vi "udp_receive_py.vi"() -> ()   [LabVIEW 2020]
panel:
  out "*(타입 *) &x":u32
  out "Numeric 4":dbl
  in  "send object cluster":T1
  in  "stop 2":bool
  out "Rz":sgl
  out "Ry":sgl
  out "Rx":sgl
  out "z":sgl
  out "y":sgl
  out "x":sgl
  out "error":sgl
  out "function":sgl
  out "string":string
  in  "stop":bool
  out "Numeric":i32
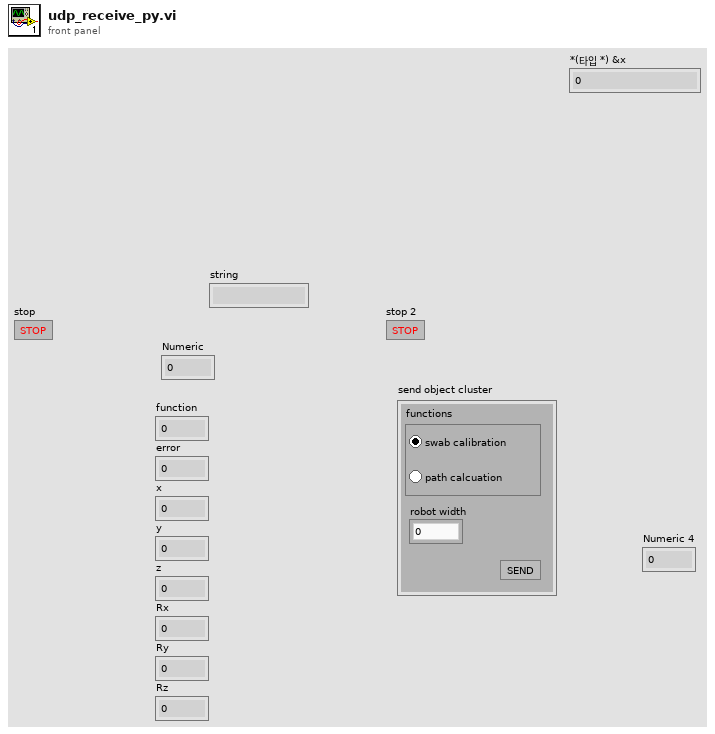
[diagram p1: front panel]
types:
  T1 = cluster{"functions":enum32{"swab calibration", "path calculation"}, "robot width":sgl, "send":bool}
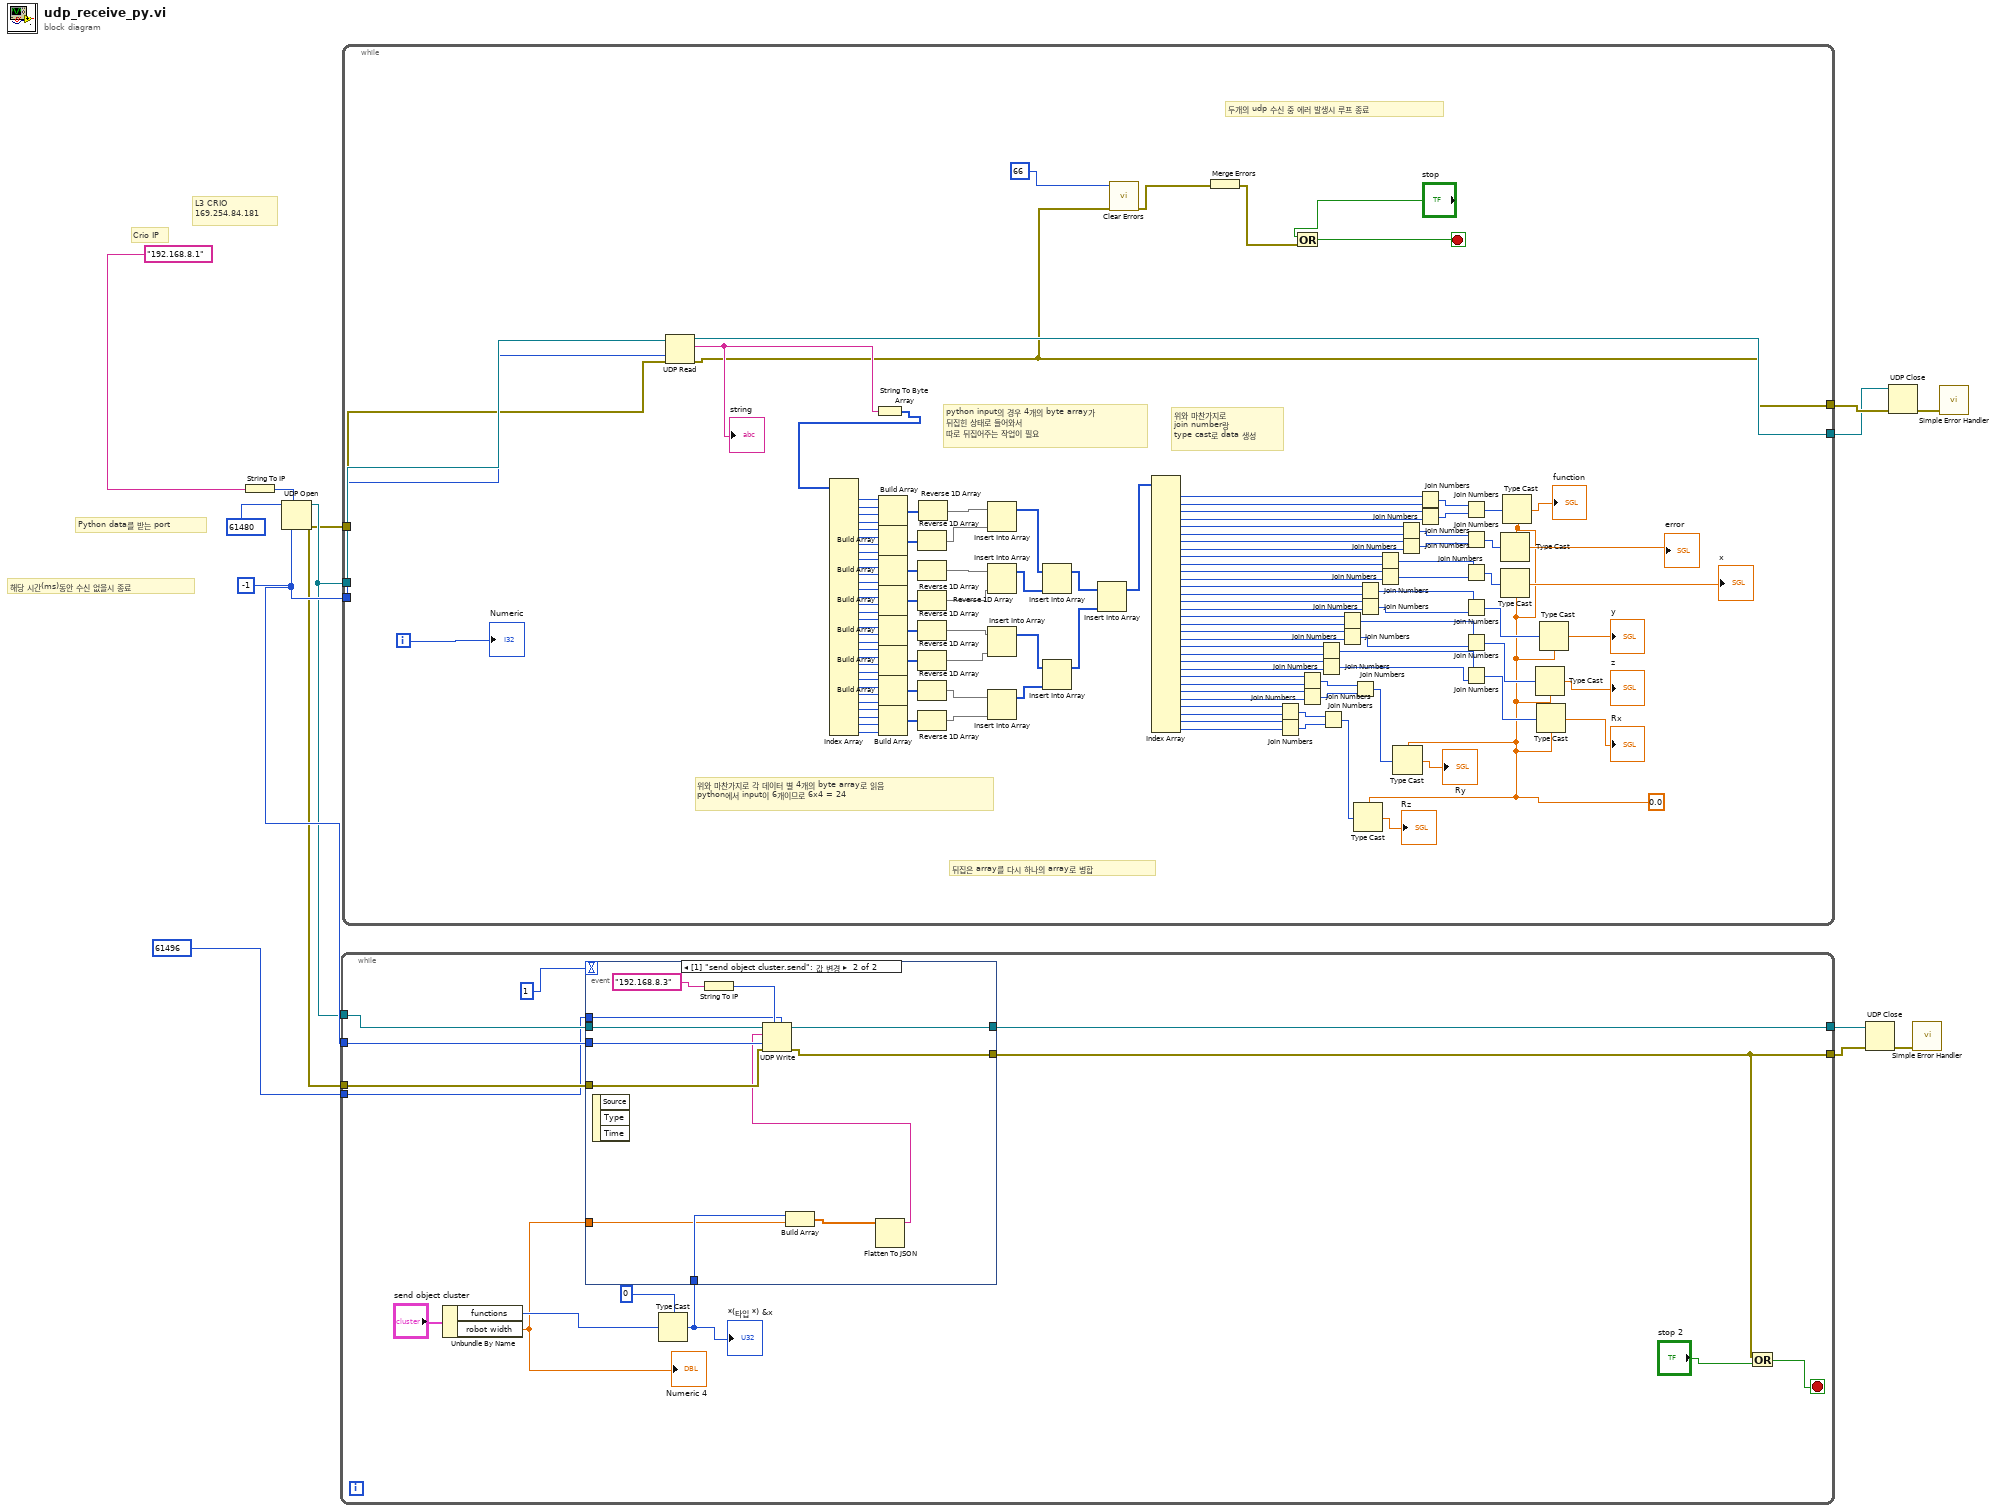
[diagram p0: block diagram]
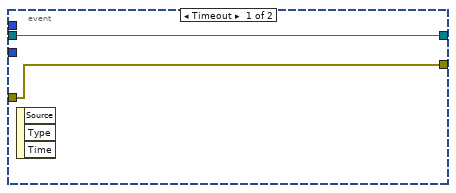
[diagram p2: hidden frame]
diagram:
  w5 = -1 ("timeout ms (25000)")
  # "L3 CRIO\n169.254.84.181"
  # "해당 시간(ms)동안 수신 없을시 종료"
  # "Crio IP"
  # "Python data를 받는 port"
  n1 = String To IP(1:"192.168.8.1" ("service name")) -> (0:w12:u32)
  n2 = UDP Open(7:w12, 9:w5, 11:u16 61480 ("port")) -> (port=w4:refnum<k16>, 0:w3:errorcluster)  [unwired: 2 in, 1 out]
  n3 = while {
    tunnel: w4 -> [w27]
    tunnel: w5 -> [w26]
    tunnel: w3 -> [w25]
    tunnel: [w24] -> w8
    tunnel: [w23] -> w7
    tunnel: u16 61496 ("port") -> [w19]
    stop <- w22 stop-if-true
    n4 = Unbundle By Name("send object cluster") -> ("functions"=w16:enum32{"swab calibration", "path calculation"}, "robot width"=w14:sgl)
    "Numeric 4" <- w14
    n5 = Type Cast(type=u32 0, x=w16) -> (*(type *) &x=w15:u32)
    "*(타입 *) &x" <- w15
    n6 = event shown="[1] \"send object cluster.send\": 값 변경" {
      selector: _ -> [_ _]
      dyn-events: _ -> [_ _]
      timeout: 1 ("timeout ms (25000)") -> [_ _]
      tunnel: w27 -> [w29 w41]
      tunnel: w26 -> [_ w40]
      tunnel: w25 -> [w28 w39]
      tunnel: [w29 w36] -> w24
      tunnel: [w28 w35] -> w23
      tunnel: w19 -> [_ w34]
      tunnel: w15 -> [_ w32]
      tunnel: w14 -> [_ w31]
      event Timeout {
        n7 = event-data() -> ()  [unwired: 1 in, 3 out]
      }
      event "send object cluster.send": Value Change {
        n8 = event-data() -> ()  [unwired: 1 in, 3 out]
        n9 = String To IP(1:"192.168.8.3" ("service name")) -> (0:w37:u32)
        n10 = Build Array(w32, w31) -> (w33:sgl[])
        n11 = Flatten To JSON(anything=w33) -> (JSON string=w30:string)  [unwired: 2 in, 1 out]
        n12 = UDP Write(address=w37, port or service name=w34, connection ID=w41, data in=w30, 8:w39, 9:w40) -> (error out=w35:errorcluster, 3:w36:refnum<k16>)
      }
    }
    n13 = Or(x=w23, y="stop 2") -> (x .or. y?=w22:bool)
  }
  n14 = while {
    tunnel: w4 -> [w171]
    tunnel: w5 -> [w170]
    tunnel: w3 -> [w169]
    tunnel: [w44] -> w11
    tunnel: [w168] -> w10
    i -> [w174]
    stop <- w172 stop-if-true
    w47 = sgl 0.0
    # "두개의 udp 수신 중 에러 발생시 루프 종료"
    # "위와 마찬가지로\njoin number랑\ntype cast로 data 생성"
    # "뒤집은 array를 다시 하나의 array로 병합"
    # "python input의 경우 4개의 byte array가\n뒤집힌 상태로 들어와서\n따로 뒤집어주는 작업이 필요"
    # "위와 마찬가지로 각 데이터 별 4개의 byte array로 읽음\npython에서 input이 6개이므로 6x4 = 24"
    n15 = UDP Read(connection ID=w171, timeout ms (25000)=w170, 8:w169) -> (data out=w131:string, error out=w44:errorcluster, 3:w168:refnum<k16>)  [unwired: 1 in, 2 out]
    "string" <- w131
    n16 = String To Byte Array(string=w131) -> (unsigned byte array=w165:u8[])
    n17 = Index Array(array=w165) -> (element #1=w166:u8, element #2=w164:u8, element #3=w163:u8, element #4=w162:u8, element #5=w161:u8, element #6=w160:u8, element #7=w159:u8, element #8=w158:u8, element #9=w157:u8, element #10=w156:u8, element #11=w155:u8, element #12=w154:u8, element #13=w130:u8, element #14=w129:u8, element #15=w128:u8, element #16=w127:u8, element #17=w126:u8, element #18=w125:u8, element #19=w124:u8, element #20=w123:u8, element #21=w122:u8, element #22=w121:u8, element #23=w120:u8, element #24=w119:u8, element #25=w88:u8, element #26=w87:u8, element #27=w86:u8, element #28=w85:u8, element #29=w84:u8, element #30=w83:u8, element #31=w82:u8, element #32=w81:u8)  [unwired: 32 in]
    n18 = Build Array(w166, w164, w163, w162) -> (w153:u8[])
    n19 = Build Array(w161, w160, w159, w158) -> (w152:u8[])
    n20 = Build Array(w157, w156, w155, w154) -> (w151:u8[])
    n21 = Build Array(w130, w129, w128, w127) -> (w118:u8[])
    n22 = Build Array(w126, w125, w124, w123) -> (w117:u8[])
    n23 = Build Array(w122, w121, w120, w119) -> (w116:u8[])
    n24 = Build Array(w88, w87, w86, w85) -> (w80:u8[])
    n25 = Build Array(w84, w83, w82, w81) -> (w79:u8[])
    n26 = Reverse 1D Array(array=w152) -> (reversed array=w149:u8[])
    n27 = Reverse 1D Array(array=w151) -> (reversed array=w115:u8[])
    n28 = Reverse 1D Array(array=w118) -> (reversed array=w114:u8[])
    n29 = Reverse 1D Array(array=w117) -> (reversed array=w113:u8[])
    n30 = Reverse 1D Array(array=w116) -> (reversed array=w112:u8[])
    n31 = Reverse 1D Array(array=w80) -> (reversed array=w78:u8[])
    n32 = Reverse 1D Array(array=w79) -> (reversed array=w77:u8[])
    n33 = Reverse 1D Array(array=w153) -> (reversed array=w150:u8[])
    n34 = Insert Into Array(array=w150, new element=w149) -> (w74:u8[])  [unwired: 1 in]
    n35 = Insert Into Array(array=w115, new element=w114) -> (w73:u8[])  [unwired: 1 in]
    n36 = Insert Into Array(array=w113, new element=w112) -> (w75:u8[])  [unwired: 1 in]
    n37 = Insert Into Array(array=w78, new element=w77) -> (w76:u8[])  [unwired: 1 in]
    n38 = Insert Into Array(array=w74, new element=w73) -> (w72:u8[])  [unwired: 1 in]
    n39 = Insert Into Array(array=w75, new element=w76) -> (w71:u8[])  [unwired: 1 in]
    n40 = Insert Into Array(array=w72, new element=w71) -> (w148:u8[])  [unwired: 1 in]
    n41 = call <vilib>:"Clear Errors.vi"("error in (no error)"=w44, "specific error code to clear (0: all)"=66) -> ("error out"=w43:errorcluster)  [unwired: 4 in, 1 out]
    n42 = Index Array(array=w148) -> (element #1=w146:u8, element #2=w145:u8, element #3=w144:u8, element #4=w143:u8, element #5=w142:u8, element #6=w98:u8, element #7=w147:u8, element #8=w97:u8, element #9=w141:u8, element #10=w94:u8, element #11=w93:u8, element #12=w92:u8, element #13=w107:u8, element #14=w91:u8, element #15=w90:u8, element #16=w89:u8, element #17=w70:u8, element #18=w69:u8, element #19=w68:u8, element #20=w67:u8, element #21=w106:u8, element #22=w65:u8, element #23=w64:u8, element #24=w63:u8, element #25=w61:u8, element #26=w60:u8, element #27=w59:u8, element #28=w58:u8, element #29=w57:u8, element #30=w56:u8, element #31=w55:u8, element #32=w54:u8)  [unwired: 32 in]
    n43 = Merge Errors(w43) -> (w167:errorcluster)
    n44 = Join Numbers(hi=w57, lo=w56) -> ((hi.lo)=w53:u16)
    n45 = Join Numbers(hi=w55, lo=w54) -> ((hi.lo)=w52:u16)
    n46 = Or(x="stop", y=w167) -> (x .or. y?=w172:bool)
    n47 = Join Numbers(hi=w61, lo=w60) -> ((hi.lo)=w51:u16)
    n48 = Join Numbers(hi=w59, lo=w58) -> ((hi.lo)=w50:u16)
    n49 = Join Numbers(hi=w106, lo=w65) -> ((hi.lo)=w108:u16)
    n50 = Join Numbers(hi=w64, lo=w63) -> ((hi.lo)=w62:u16)
    n51 = Join Numbers(hi=w53, lo=w52) -> ((hi.lo)=w49:u32)
    n52 = Join Numbers(hi=w70, lo=w69) -> ((hi.lo)=w109:u16)
    n53 = Join Numbers(hi=w68, lo=w67) -> ((hi.lo)=w66:u16)
    n54 = Join Numbers(hi=w51, lo=w50) -> ((hi.lo)=w48:u32)
    n55 = Type Cast(type=w47, x=w49) -> (*(type *) &x=→"Rz":sgl)
    n56 = Join Numbers(hi=w107, lo=w91) -> ((hi.lo)=w110:u16)
    n57 = Join Numbers(hi=w90, lo=w89) -> ((hi.lo)=w111:u16)
    n58 = Join Numbers(hi=w141, lo=w94) -> ((hi.lo)=w139:u16)
    n59 = Join Numbers(hi=w93, lo=w92) -> ((hi.lo)=w138:u16)
    n60 = Type Cast(type=w47, x=w48) -> (*(type *) &x=→"Ry":sgl)
    n61 = Join Numbers(hi=w142, lo=w98) -> ((hi.lo)=w96:u16)
    n62 = Join Numbers(hi=w147, lo=w97) -> ((hi.lo)=w95:u16)
    n63 = Join Numbers(hi=w146, lo=w145) -> ((hi.lo)=w99:u16)
    n64 = Join Numbers(hi=w144, lo=w143) -> ((hi.lo)=w140:u16)
    n65 = Join Numbers(hi=w99, lo=w140) -> ((hi.lo)=w136:u32)
    n66 = Join Numbers(hi=w96, lo=w95) -> ((hi.lo)=w135:u32)
    n67 = Join Numbers(hi=w139, lo=w138) -> ((hi.lo)=w137:u32)
    n68 = Join Numbers(hi=w110, lo=w111) -> ((hi.lo)=w105:u32)
    n69 = Join Numbers(hi=w109, lo=w66) -> ((hi.lo)=w104:u32)
    n70 = Join Numbers(hi=w108, lo=w62) -> ((hi.lo)=w103:u32)
    n71 = Type Cast(type=w47, x=w135) -> (*(type *) &x=→"error":sgl)
    n72 = Type Cast(type=w47, x=w137) -> (*(type *) &x=→"x":sgl)
    n73 = Type Cast(type=w47, x=w136) -> (*(type *) &x=→"function":sgl)
    n74 = Type Cast(type=w47, x=w104) -> (*(type *) &x=→"z":sgl)
    n75 = Type Cast(type=w47, x=w103) -> (*(type *) &x=→"Rx":sgl)
    n76 = Type Cast(type=w47, x=w105) -> (*(type *) &x=→"y":sgl)
    "Numeric" <- w174
  }
  n77 = UDP Close(connection ID=w8, 8:w7) -> (error out=w6:errorcluster)  [unwired: 1 out]
  n78 = UDP Close(connection ID=w10, 8:w11) -> (error out=w1:errorcluster)  [unwired: 1 out]
  n79 = call <vilib>:"Simple Error Handler.vi"("error in (no error)"=w6) -> ()  [unwired: 4 in, 5 out]
  n80 = call <vilib>:"Simple Error Handler.vi"("error in (no error)"=w1) -> ()  [unwired: 4 in, 5 out]
